vi "Globals.vi"() -> ()   [LabVIEW 2014]
panel:
  out "Degrees":dbl
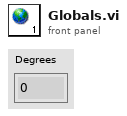
[diagram p1: front panel]
diagram:
